vi "Get Angles.vi"(8 "error in (no error)":errorcluster, 11 "Inclinometer in":refnum<class "Inclinometer.lvclass">) -> (0 "error out":errorcluster, 2 "Angles":dbl[](array[numeric]), 3 "Inclinometer out":refnum<class "Inclinometer.lvclass">)   [LabVIEW 2016, in "Hardware.lvlib" / "Inclinometer.lvlib" / "Inclinometer.lvclass"]
uses:
  <userlib>/Common Components/Hardware/Inclinometer/Inclinometer/Inclinometer.lvclass
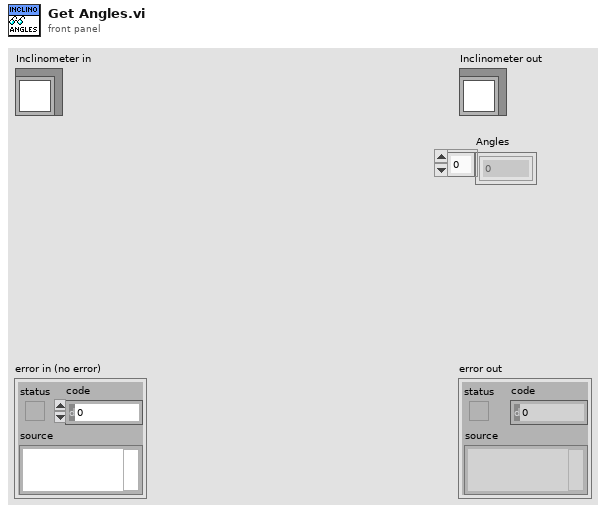
[diagram p1: front panel]
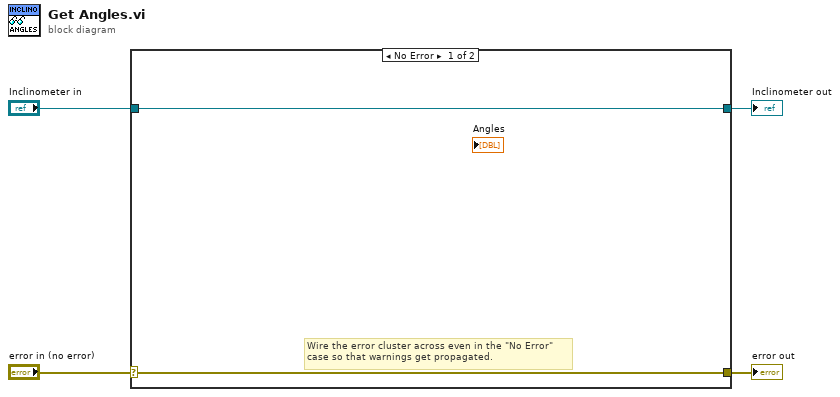
[diagram p0: block diagram]
diagram:
  n1 = case shown="No Error" "error in (no error)" {
    selector: "error in (no error)" -> [w5 w8]
    tunnel: [w5 w8] -> w3
    tunnel: [w6 w7] -> w1
    tunnel: "Inclinometer in" -> [w6 w7]
    frame No Error {
      # "Wire the error cluster across even in the \"No Error\"\ncase so that warnings get propagated."
    }
    frame Error {
    }
  }
  "error out" <- w3
  "Inclinometer out" <- w1
